vi "whatMotorIs.vi"(5 "Device in":refnum<k24>) -> (1 "SerialNumber":u32, 2 "Device out":refnum<k24>)   [LabVIEW 2014]
doc: "André Romero - 2017\nandretec@ifsc.usp.br"
uses:
  C:/users-lab/Andre/GITs/andretec/Thorlabs-Vector-Move/kinesisTec/Kinesis/Thorlabs.MotionControl.TCube.DCServoCLI.dll
  Kinesis/Thorlabs.MotionControl.TCube.DCServoCLI.dll
  C:/users-lab/Andre/GITs/andretec/Thorlabs-Vector-Move/kinesisTec/Kinesis/Thorlabs.MotionControl.DeviceManagerCLI.dll
  Kinesis/Thorlabs.MotionControl.DeviceManagerCLI.dll
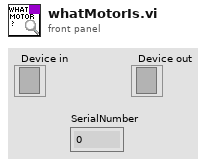
[diagram p1: front panel]
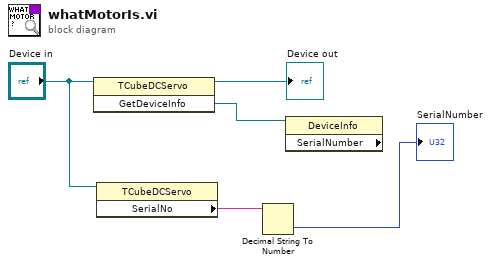
[diagram p0: block diagram]
diagram:
  n1 = invoke class="TCubeDCServo" method="GetDeviceInfo"(reference="Device in") -> (reference out=→"Device out":refnum<k24>, "GetDeviceInfo"=w4:refnum<k24>)  [unwired: 2 in, 1 out]
  n2 = property class="TCubeDCServo"(reference="Device in") -> ("SerialNo"=w2:string)  [unwired: 1 in, 2 out]
  n3 = Decimal String To Number(string=w2) -> (number=→"SerialNumber":i32)  [unwired: 2 in, 1 out]
  n4 = property class="DeviceInfo" props=["SerialNumber"](reference=w4) -> ()  [unwired: 1 in, 3 out]
